vi "rec_random.vi"() -> ()   [LabVIEW 2013]
uses:
  Global.vi
panel:
  in  "name":string="RAND"
  out "number (0 to 1)":dbl
  in  "stop":bool
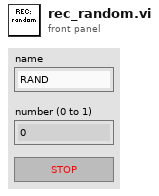
[diagram p1: front panel]
types:
  T1 = typedef "Semaphore RefNum" = refnum<k1>
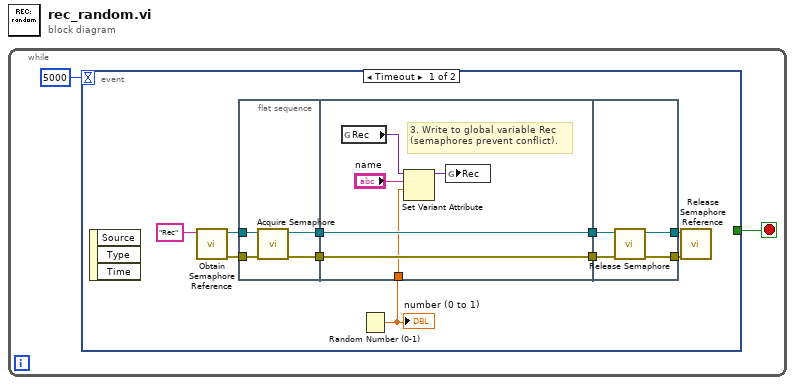
[diagram p0: block diagram]
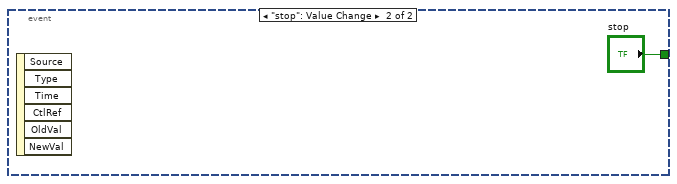
[diagram p2: hidden frame]
diagram:
  n1 = while {
    stop <- w2 stop-if-true
    n2 = event shown="[0] Timeout" {
      selector: _ -> [_ _]
      dyn-events: _ -> [_ _]
      timeout: 5000 -> [_ _]
      tunnel: [_ "stop"] -> w2
      event Timeout {
        n3 = event-data() -> ()  [unwired: 1 in, 3 out]
        n4 = call <vilib>:"Obtain Semaphore Reference.vi"("name (unnamed)"="Rec") -> ("error out"=w10:errorcluster, "semaphore"=w11:T1)  [unwired: 4 in, 1 out]
        n5 = flat-sequence {
          tunnel: w11 -> [w16]
          tunnel: w10 -> [w13]
          tunnel: [w15] -> w8
          tunnel: [w14] -> w4
          tunnel: [w22] -> w9
          tunnel: w8 -> [w22]
          tunnel: [w21] -> w5
          tunnel: w4 -> [w21]
          tunnel: w3 -> [w18]
          tunnel: w9 -> [w26]
          tunnel: [w25] -> w7
          tunnel: [w24] -> w6
          tunnel: w5 -> [w23]
          frame #0 {
            n6 = call <vilib>:"Acquire Semaphore.vi"("error in (no error)"=w13, "semaphore"=w16) -> ("error out"=w14:errorcluster, "semaphore out"=w15:T1)  [unwired: 3 in, 1 out]
          }
          frame #1 {
            # "3. Write to global variable Rec\n(semaphores prevent conflict)."
            n7 = global read "Global.vi" "Rec"() -> (w20:variant)
            n8 = Set Variant Attribute(Variant=w20, name="name", value=w18) -> (Variant out=w19:variant)  [unwired: 1 in, 2 out]
            n9 = global write "Global.vi" "Rec"(w19) -> ()
          }
          frame #2 {
            n10 = call <vilib>:"Release Semaphore.vi"("error in (no error)"=w23, "semaphore"=w26) -> ("error out"=w24:errorcluster, "semaphore out"=w25:T1)  [unwired: 4 in]
          }
        }
        n11 = Random Number (0-1)() -> (number: 0 to 1=w3:dbl)
        "number (0 to 1)" <- w3
        n12 = call <vilib>:"Release Semaphore Reference.vi"("error in (no error)"=w6, "semaphore"=w7) -> ()  [unwired: 8 in, 2 out]
      }
      event "stop": Value Change {
        n13 = event-data() -> ()  [unwired: 1 in, 6 out]
      }
    }
  }
